vi "API Example - Add.vi"(10 "input2":dbl, 11 "input1":dbl) -> (3 "sum":dbl)   [LabVIEW 2020]
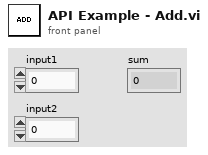
[diagram p1: front panel]
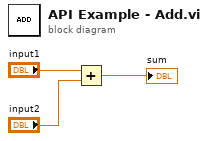
[diagram p0: block diagram]
diagram:
  n1 = Add(x="input1", y="input2") -> (x+y=→"sum":dbl)
